vi "Set Relay Command.vi"(8 "error in":errorcluster, 11 "Desired Relay State":bool[](array[boolean])) -> (0 "error out":errorcluster, 3 "connection ID":refnum<k5>)   [LabVIEW 2025, in "SafetyLight.lvlib"]
uses:
  SafetyLight.lvlib
panel:
  out "data out":string
  out "concatenated string":string
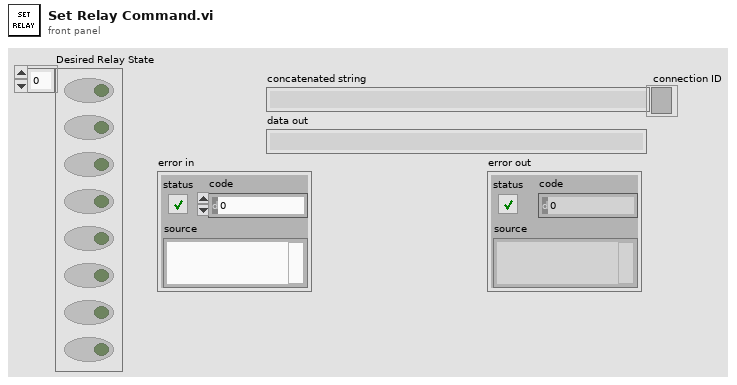
[diagram p1: front panel]
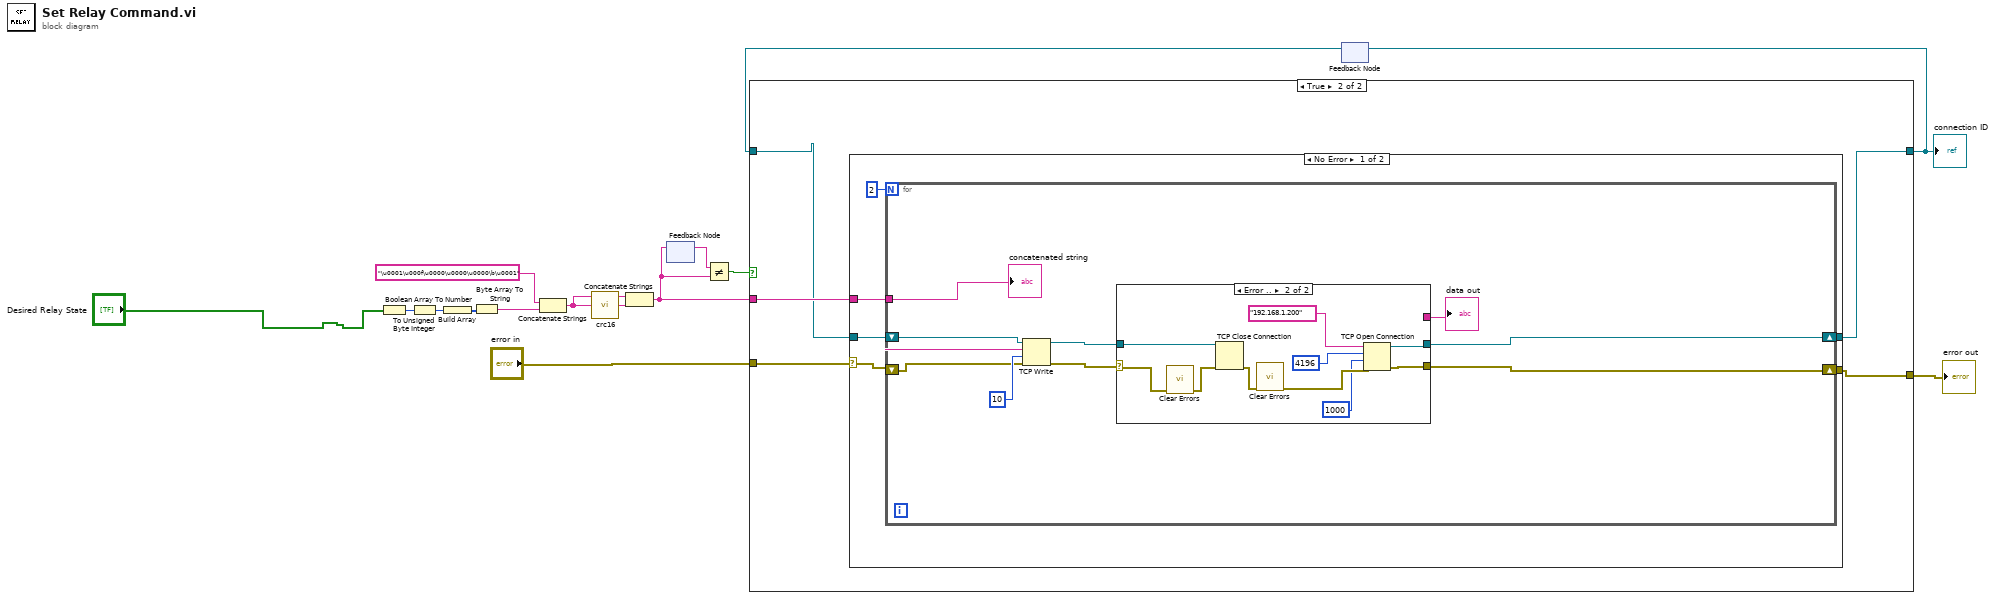
[diagram p0: block diagram]
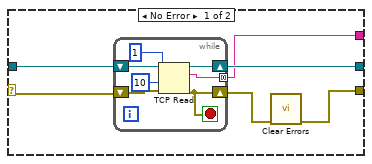
[diagram p3: hidden frame]
diagram:
  n1 = Boolean Array To Number(Boolean array="Desired Relay State") -> (number=w14:u32)
  n2 = To Unsigned Byte Integer(number=w14) -> (unsigned 8bit integer=w9:u8)
  n3 = Build Array(w9) -> (w13:u8[])
  n4 = Byte Array To String(unsigned byte array=w13) -> (string=w12:string)
  n5 = Concatenate Strings("\u0001\u000f\u0000\u0000\u0000\b\u0001" ("data in"), w12) -> (w11:string)
  n6 = call "crc16.vi"("message"=w11) -> ("CRC16"=w10:string)  [unwired: 4 in]
  n7 = Concatenate Strings(w11, w10) -> (w6:string)
  n8 = feedback-in #1(w6) -> ()
  n9 = feedback #1() -> (w5:string)  [unwired: 1 in]
  n10 = Not Equal?(x=w5, y=w6) -> (x != y?=w7:bool)
  n11 = feedback #2() -> (w3:refnum<k5>)  [unwired: 1 in]
  n12 = case shown="True" w7 {
    tunnel: [w16 w21] -> w4
    tunnel: "error in" -> [_ w18]
    tunnel: w6 -> [_ w20]
    tunnel: w3 -> [w16 w19]
    tunnel: [_ w17] -> w2
    frame False {
    }
    frame True {
      n13 = case shown="No Error" w18 {
        selector: w18 -> [w23 w61]
        tunnel: [w26 w60] -> w21
        tunnel: w20 -> [w25 _]
        tunnel: w19 -> [w24 w60]
        tunnel: [w22 w61] -> w17
        frame No Error {
          n14 = for {
            N: 2 -> [_]
            tunnel: w25 -> [w35]
            shift-right: [w28] -> w26
            shift-left: w24 -> [w36]
            shift-right: [w30] -> w22
            shift-left: w23 -> [w29]
            n15 = TCP Write(connection ID=w36, data in=w35, error in (no error)=w29, 9:10 ("timeout ms (25000)")) -> (connection ID out=w34:refnum<k5>, error out=w31:errorcluster)  [unwired: 1 out]
            n16 = case shown="Error .." w31 {
              selector: w31 -> [w37 w54]
              tunnel: w34 -> [w42 w57]
              tunnel: [w41 w56] -> w28
              tunnel: [w39 _] -> w32
              tunnel: [w38 w55] -> w30
              frame No Error {
                n17 = while {
                  shift-right: [w44] -> w40
                  shift-left: w37 -> [w49]
                  shift-right: [w47] -> w41
                  shift-left: w42 -> [w48]
                  tunnel: [w43] -> w39 mode=concatenating
                  stop <- w44 stop-if-true
                  n18 = TCP Read(connection ID=w48, bytes to read=1, error in (no error)=w49, 9:10 ("timeout ms (25000)")) -> (connection ID out=w47:refnum<k5>, data out=w43:string, error out=w44:errorcluster)  [unwired: 1 in]
                }
                n19 = call <vilib>:"Clear Errors.vi"("error in (no error)"=w40) -> ("error out"=w38:errorcluster)  [unwired: 5 in, 1 out]
              }
              frame Error {
                n20 = call <vilib>:"Clear Errors.vi"("error in (no error)"=w54) -> ("error out"=w53:errorcluster)  [unwired: 5 in, 1 out]
                n21 = TCP Close Connection(connection ID=w57, error in (no error)=w53) -> (error out=w52:errorcluster)  [unwired: 1 in, 1 out]
                n22 = call <vilib>:"Clear Errors.vi"("error in (no error)"=w52) -> ("error out"=w51:errorcluster)  [unwired: 5 in, 1 out]
                n23 = TCP Open Connection(address="192.168.1.200", remote port or service name=u16 4196, timeout ms (60000)=1000, error in (no error)=w51) -> (connection ID=w56:refnum<k5>, error out=w55:errorcluster)  [unwired: 1 in]
              }
            }
            "data out" <- w32
            "concatenated string" <- w35
          }
        }
        frame Error {
        }
      }
    }
  }
  "connection ID" <- w4
  "error out" <- w2
  n24 = feedback-in #2(w4) -> ()
